vi "Graph.vi"() -> ()   [LabVIEW 2019]
panel:
  out "Boolean":bool
  in  "Start":bool
  out "Horizontal Progress Bar":i32(slide) scale=0.0..100.0
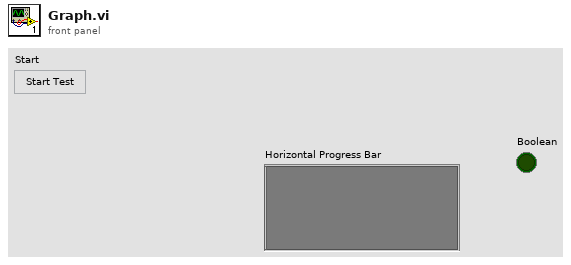
[diagram p1: front panel]
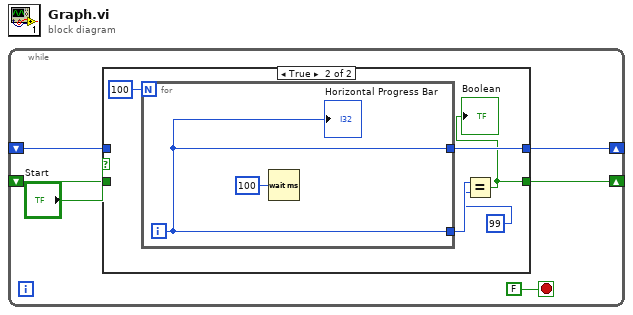
[diagram p0: block diagram]
diagram:
  n1 = while {
    shift-right: [w3] -> _
    shift-left: _ -> [w4]
    shift-right: [w1] -> _
    shift-left: _ -> [w2]
    stop <- FALSE stop-if-true
    n2 = case shown="True" "Start" {
      tunnel: [w8 w12] -> w3
      tunnel: w4 -> [w8 _]
      tunnel: [w7 w10] -> w1
      tunnel: w2 -> [w7 _]
      frame False {
      }
      frame True {
        n3 = for {
          N: 100 -> [_]
          tunnel: [w14] -> w12
          tunnel: [w14] -> w11
          i -> [w14]
          n4 = Wait (ms)(milliseconds to wait=u32 100) -> ()  [unwired: 1 out]
          "Horizontal Progress Bar" <- w14
        }
        n5 = Equal?(x=w11, y=99) -> (x = y?=w10:bool)
        "Boolean" <- w10
      }
    }
  }
